vi "Pre Launch Init.vi"(11 "工况数据UI in":refnum<class "工况数据UI.lvclass"> caption="操作者输入") -> (0 "error out":errorcluster caption="错误输出", 3 "工况数据UI out":refnum<class "工况数据UI.lvclass"> caption="操作者输出")   [LabVIEW 2016, in "工况数据UI.lvlib" / "工况数据UI.lvclass"]
doc: "(<B>Filename</B>: Actor Framework.lvlib:Actor.lvclass:Pre Launch Init.vi)\n\nDefines behavior that occurs after the Launch Nested Actor method is invoked but before the actor's Actor Core method begins running.\n\nBy default, this method does nothing.子孙类重写该方法定义具体的操作。"
uses:
  <vilib>/ActorFramework/Actor/Actor.lvclass
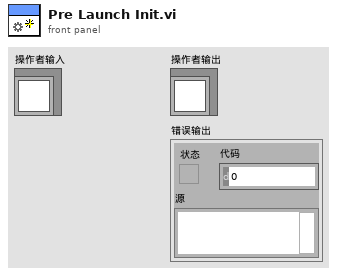
[diagram p1: front panel]
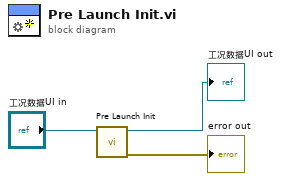
[diagram p0: block diagram]
diagram:
  n1 = call-parent "Pre Launch Init.vi"("Actor in"="工况数据UI in") -> ("error out"=→"error out":errorcluster, "Actor out"=→"工况数据UI out":refnum<class "工况数据UI.lvclass">)  [unwired: 9 in]
